vi "host-not-parelleled.vi"() -> ()   [LabVIEW 2020]
panel:
  out "max iteration":dbl
  out "iteration":dbl
  out "X":dbl[][](array[numeric])
  in  "X data filepath":path
  in  "stop":bool
  out "y waveform":cluster{"Numeric":dbl, "Double":dbl}(graph)
  out "y":dbl[][](array[numeric])
  in  "y data filepath":path
  out "Waveform Graph":dbl[][](graph)
  out "y predict values":dbl[](array[numeric])
  out "x waveform":dbl(graph)
  out "t":dbl[][](array[numeric])
  in  "t data filepath":path
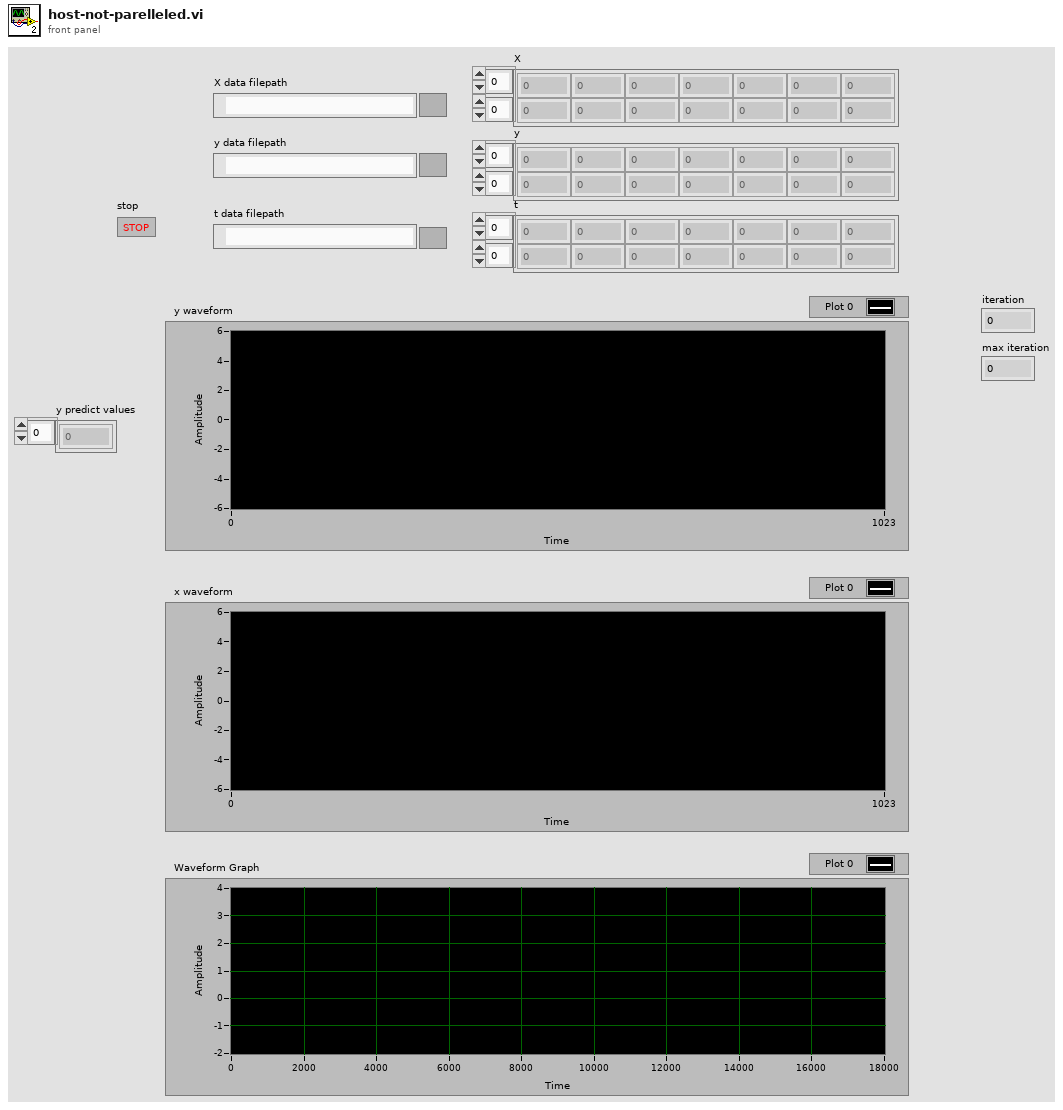
[diagram p1: front panel]
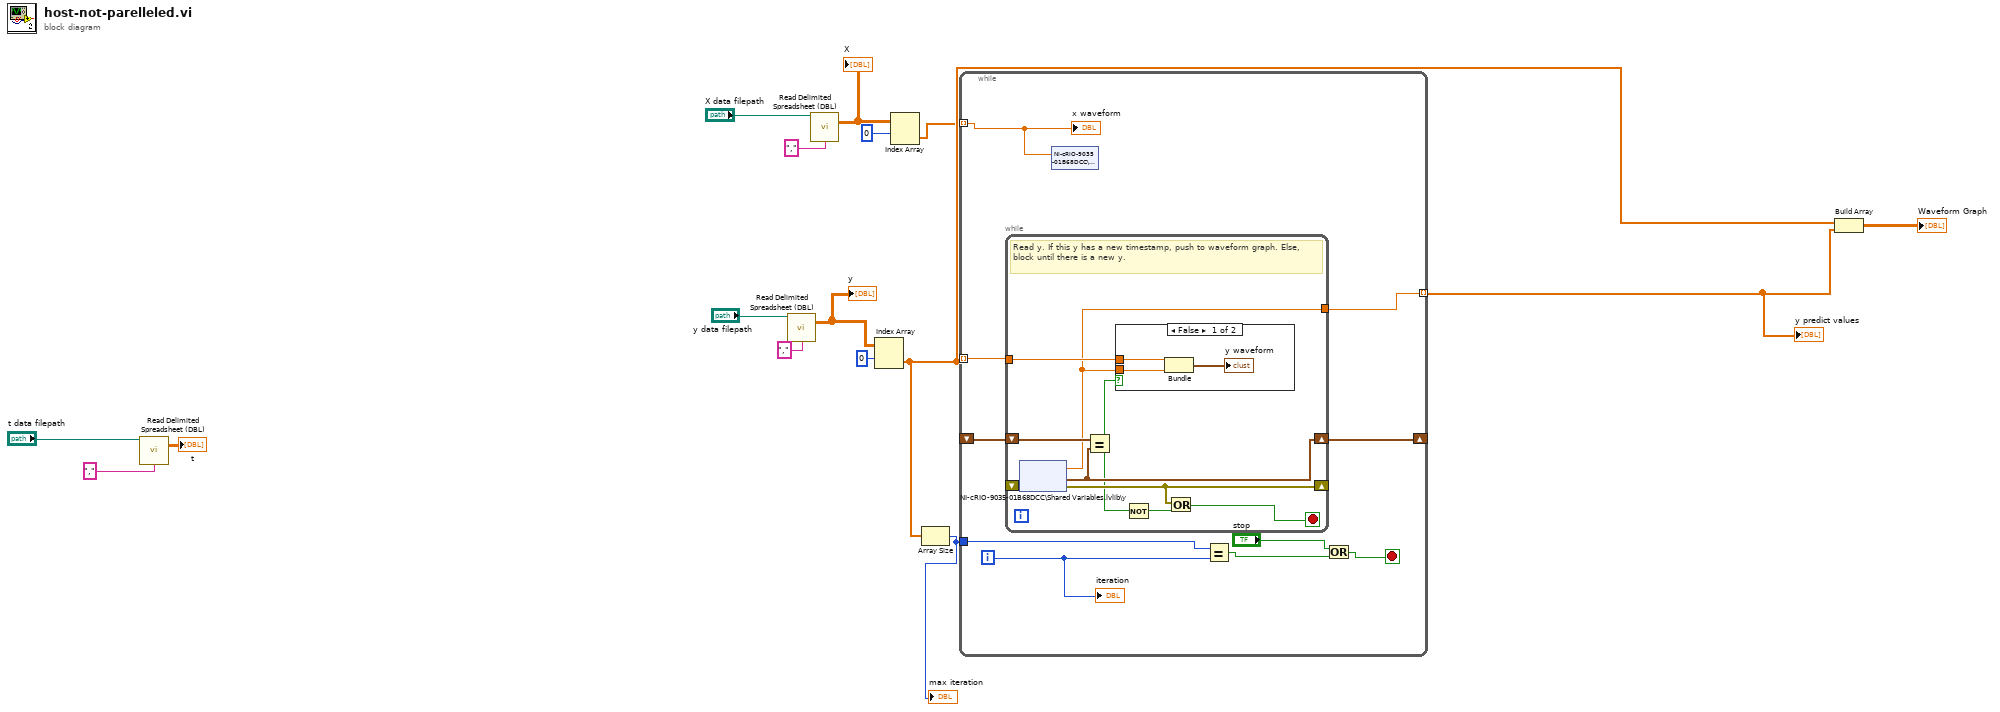
[diagram p0: block diagram]
diagram:
  n1 = call <vilib>:"Read Delimited Spreadsheet (DBL).vi"("file path (dialog if empty)"="t data filepath", "delimiter (\\t)"=",") -> ("all rows"=→"t":dbl[][])  [unwired: 8 in, 5 out]
  n2 = call <vilib>:"Read Delimited Spreadsheet (DBL).vi"("file path (dialog if empty)"="y data filepath", "delimiter (\\t)"=",") -> ("all rows"=w9:dbl[][])  [unwired: 8 in, 5 out]
  "y" <- w9
  n3 = call <vilib>:"Read Delimited Spreadsheet (DBL).vi"("file path (dialog if empty)"="X data filepath", "delimiter (\\t)"=",") -> ("all rows"=w5:dbl[][])  [unwired: 8 in, 5 out]
  "X" <- w5
  n4 = Index Array(array=w9, index (row)=0) -> (element=w3:dbl[])  [unwired: 1 in]
  n5 = Index Array(array=w5, index (row)=0) -> (element=w2:dbl[])  [unwired: 1 in]
  n6 = Array Size(array=w3) -> (size(s)=w1:i32)
  "max iteration" <- w1
  n7 = while {
    tunnel: w3 -> [w26] mode=indexing
    tunnel: [w23] -> w8 mode=indexing
    shift-right: [w25] -> _
    shift-left: _ -> [w24]
    tunnel: w1 -> [w22]
    tunnel: w2 -> [w18] mode=indexing
    i -> [w17]
    stop <- w20 stop-if-true
    n8 = while {
      shift-right: [w34] -> w25
      shift-left: w24 -> [w33]
      shift-right: [w32] -> _
      shift-left: _ -> [w35]
      tunnel: w26 -> [w29]
      tunnel: [w28] -> w23
      stop <- w27 stop-if-true
      # "Read y. If this y has a new timestamp, push to waveform graph. Else, block until there is a new y."
      n9 = shared-variable "NI-cRIO-9035-01B68DCC\\Shared Variables.lvlib\\y"(error in=w35) -> (w28:dbl, error out=w32:errorcluster, w34:timestamp)
      n10 = Equal?(x=w33, y=w34) -> (x = y?=w30:bool)
      n11 = case shown="False" w30 {
        tunnel: w29 -> [w37 _]
        tunnel: w28 -> [w36 _]
        frame False {
          n12 = Bundle("Numeric"=w37, "Double"=w36) -> (→"y waveform":cluster{"Numeric":dbl, "Double":dbl})  [unwired: 1 in]
        }
        frame True {
        }
      }
      n13 = Not(x=w30) -> (.not. x?=w31:bool)
      n14 = Or(x=w32, y=w31) -> (x .or. y?=w27:bool)
    }
    n15 = shared-variable "NI-cRIO-9035-01B68DCC\\Shared Variables.lvlib\\x"(w18) -> ()  [unwired: 1 in, 1 out]
    n16 = Equal?(x=w22, y=w17) -> (x = y?=w19:bool)
    n17 = Or(x="stop", y=w19) -> (x .or. y?=w20:bool)
    "x waveform" <- w18
    "iteration" <- w17
  }
  "y predict values" <- w8
  n18 = Build Array(w3, w8) -> (→"Waveform Graph":dbl[][])
